vi "Reference Facade.vi"(0 "Data In":T4, 2 "Display State In":T2, 3 "Container State":T3) -> (6 "Data Out":T4, 7 "Display State Out":T2, 8 "Action":T1)   [LabVIEW 2016, in "VI Reference.xctl"]
uses:
  VI Reference.xctl
  Reference Data.ctl
  <vilib>/_xctls/Container State.ctl
  Reference State.ctl
  VI Reference Control/VI Reference Control.lvclass
  C:/Users/tblair/Documents/Git Projects/Drag and Drop VI Tool/Source/Reference Control/Reference Control.lvclass
  <vilib>/_xctls/Action.ctl
  <vilib>/Utility/miscctls.llb/LVRectTypeDef.ctl
  <vilib>/_xctls/XControlSupport.lvlib
  Reference Control/Reference Control.lvclass
panel:
  in  "Source Path":path
  out "Source Picture":picture
  # "1. Drop the controls that make up the appearance\nof the XControl here.\n\n2. Resize the window to fit the controls\n\n3. If the XControl is of fixed size,  make the \n window not resizable from VI Properties->Window Appearance.\n\n4. If you want the controls to automatically size when the XControl sizes, check  \"Scale all objects on front panel when window resizes\" in File->VI Properties->Window Size page.\n\n5. Show the block diagram and handle events for the controls on this panel."
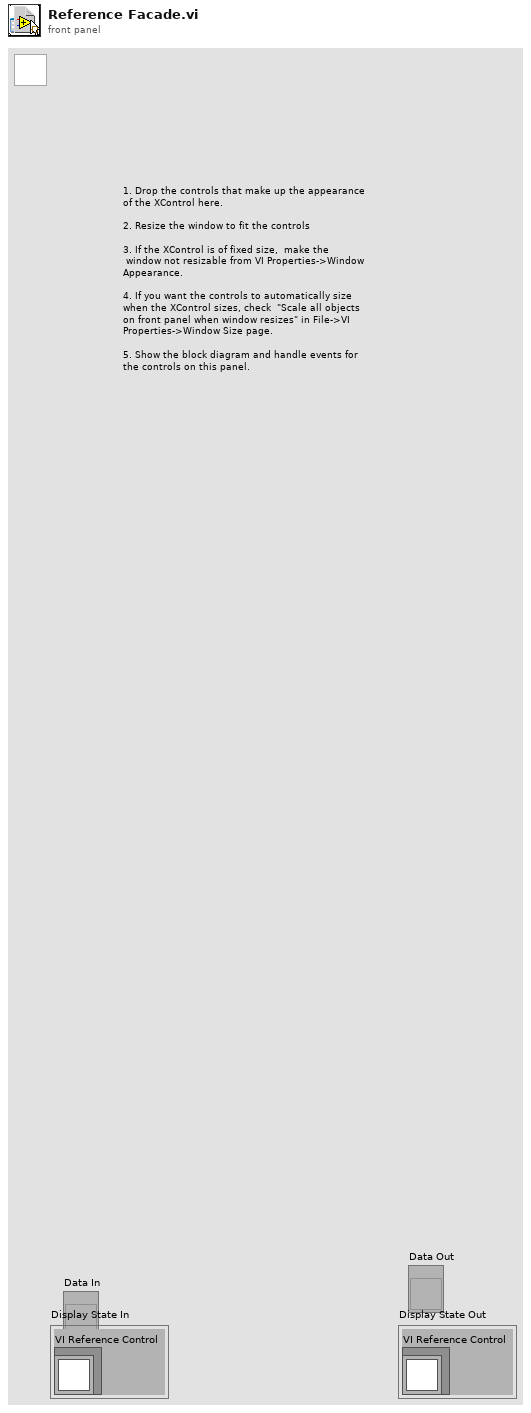
[diagram p1: front panel]
types:
  T1 = typedef "XControlSupport.lvlib/Action.ctl" = cluster{"Data Changed?":bool, "State Changed?":bool, "Action Name":string}
  T2 = typedef "VI Reference.xctl/Reference State.ctl" = cluster{"VI Reference Control":refnum<class "VI Reference Control.lvclass">}
  T3 = typedef "XControlSupport.lvlib/Container State.ctl" = cluster{"Indicator?":bool, "Run Mode?":bool, " Refnum":refnum<vi>}
  T4 = typedef "VI Reference.xctl/Reference Data.ctl" = refnum<vi>
  T5 = typedef "LVRectTypeDef.ctl" = cluster{"Left":i16, "Top":i16, "Right":i16, "Bottom":i16}
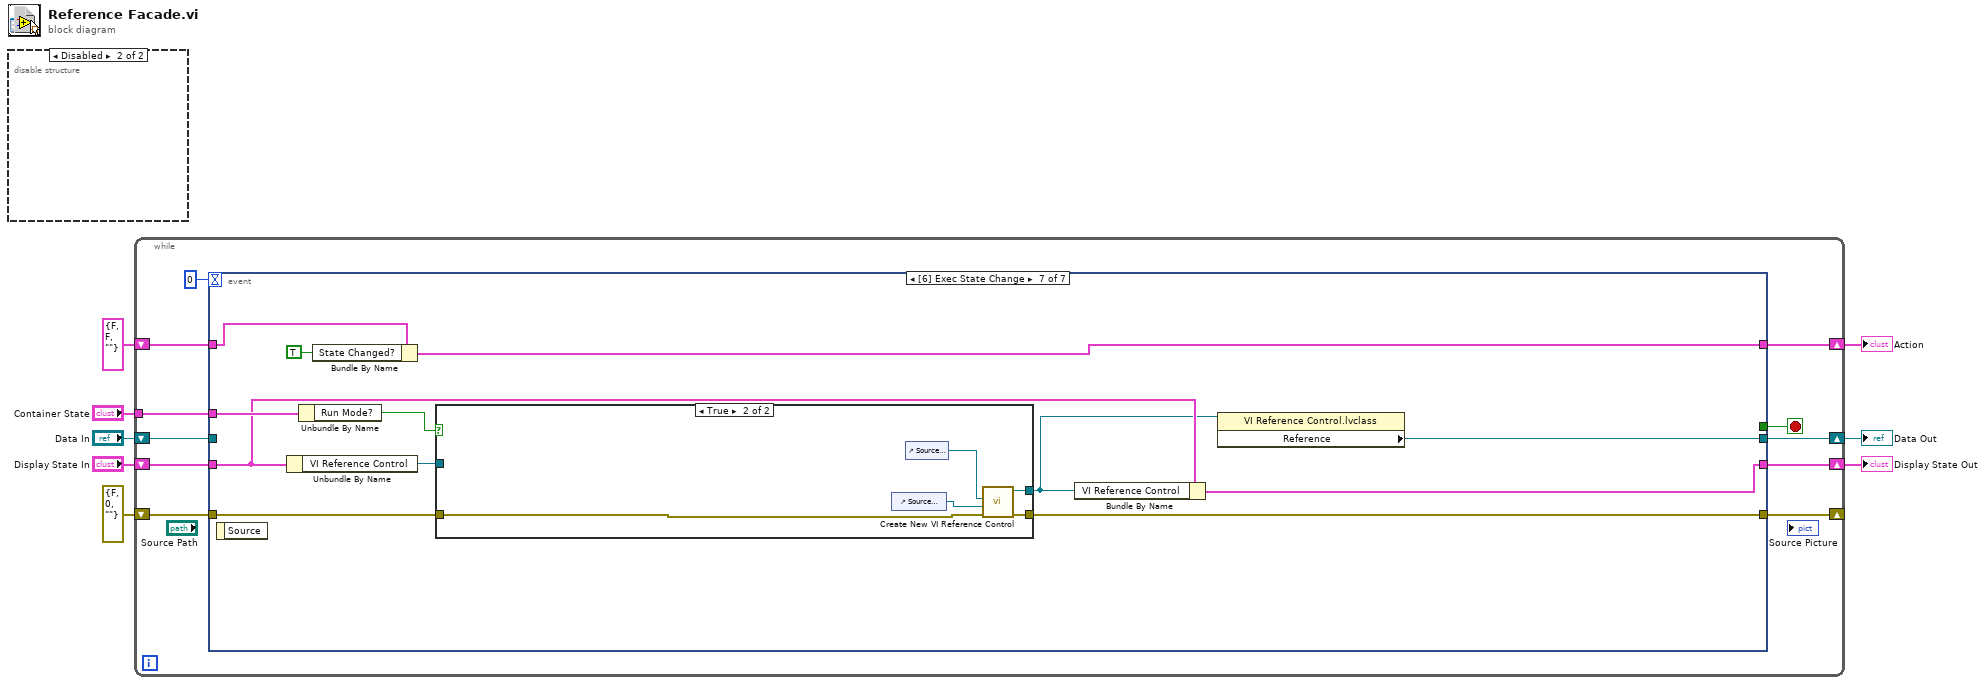
[diagram p0: block diagram]
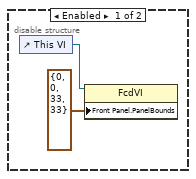
[diagram p2: hidden frame]
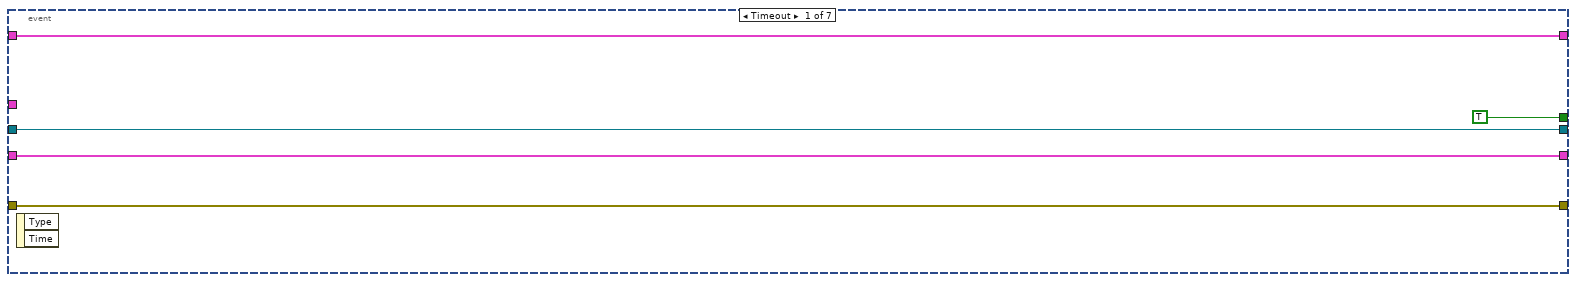
[diagram p3: hidden frame]
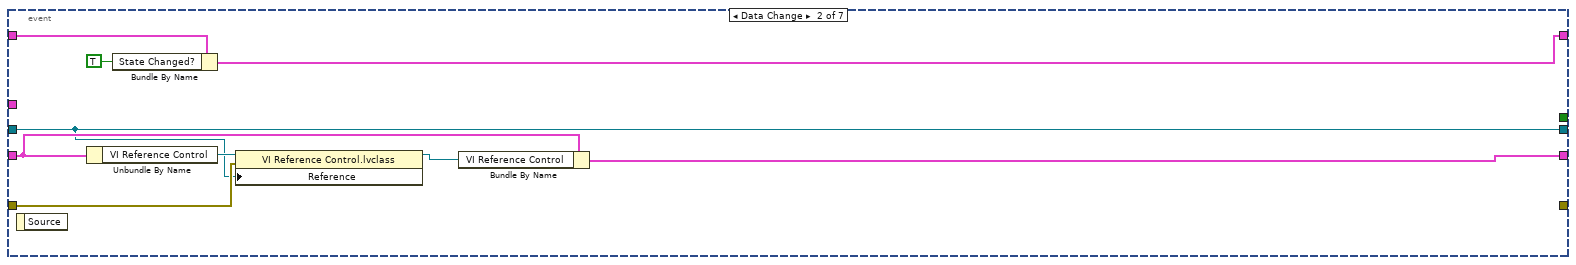
[diagram p4: hidden frame]
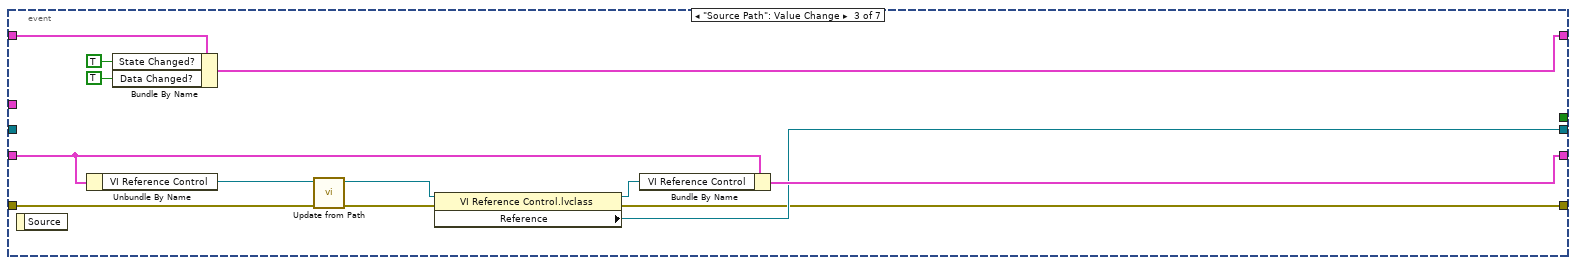
[diagram p5: hidden frame]
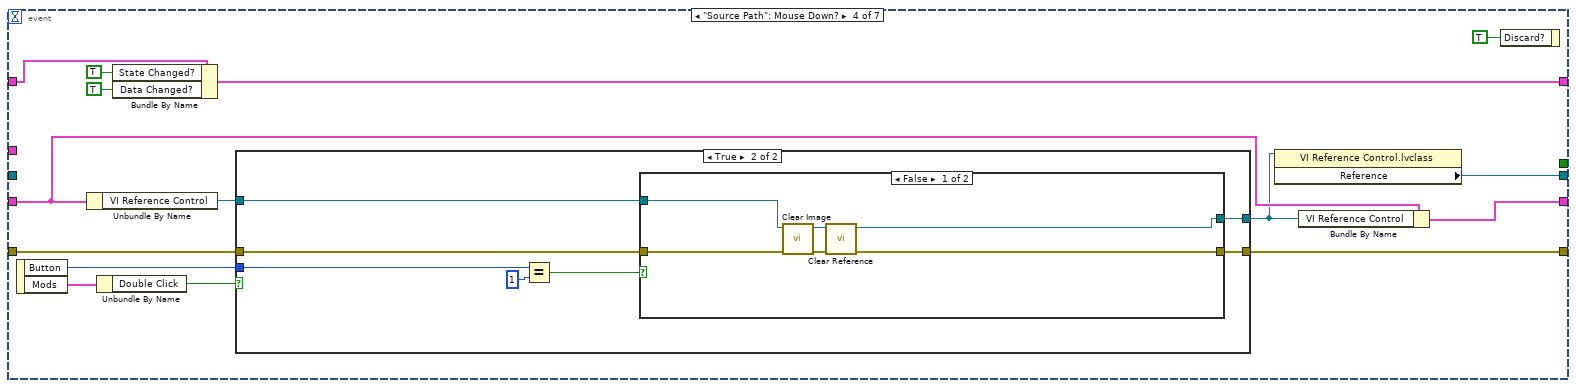
[diagram p6: hidden frame]
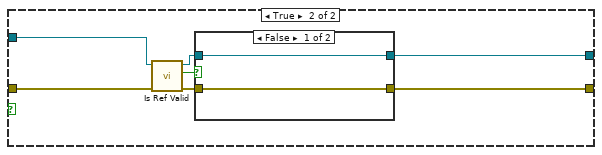
[diagram p8: hidden frame]
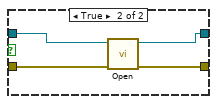
[diagram p9: hidden frame]
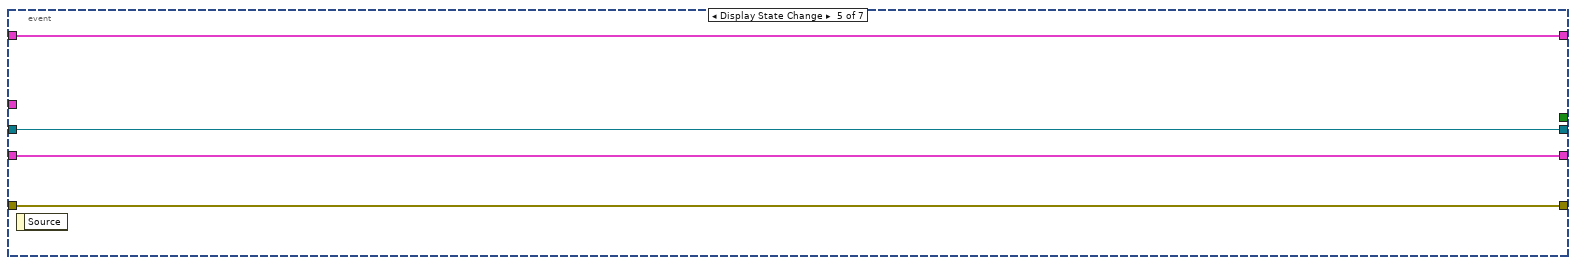
[diagram p10: hidden frame]
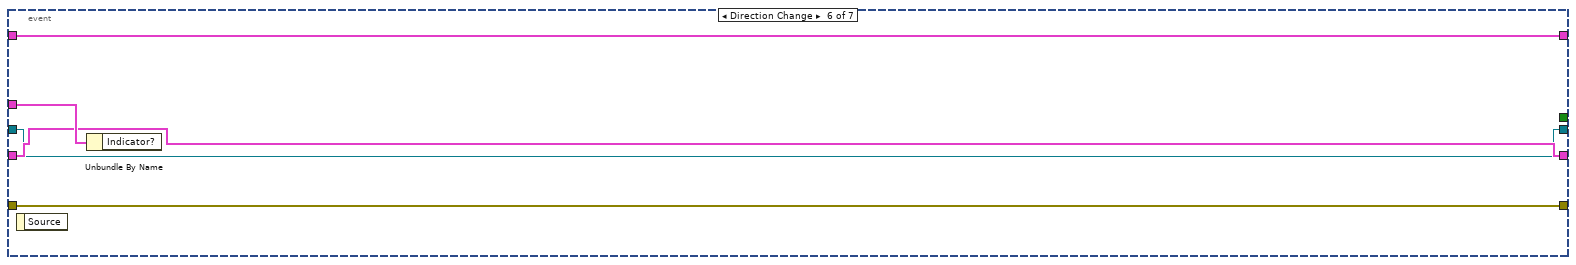
[diagram p11: hidden frame]
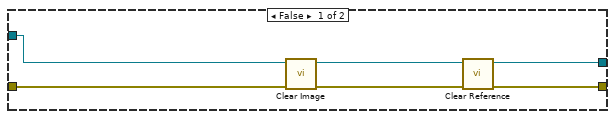
[diagram p12: hidden frame]
diagram:
  n1 = disable-structure shown="Disabled" {
    frame Enabled {
      n2 = control-ref of="This VI"() -> (w9:refnum<vi>)
      n3 = property class="FcdVI"(reference=w9, "Front Panel.PanelBounds"=T5 {"Left"=0, "Top"=0, "Right"=33, "Bottom"=33} ("Front Panel Window:Panel Bounds")) -> ()  [unwired: 1 in, 2 out]
    }
    frame Disabled {
    }
  }
  n4 = while {
    shift-right: [w20] -> w6
    shift-left: "Display State In" -> [w21]
    tunnel: "Container State" -> [w17]
    shift-right: [w15] -> w1
    shift-left: "Data In" -> [w16]
    shift-right: [w13] -> w4
    shift-left: T1 {"Data Changed?"=FALSE, "State Changed?"=FALSE, "Action Name"=""} ("Action") -> [w14]
    shift-right: [w12] -> _
    shift-left: errorcluster {"status"=FALSE, "code"=0, "source"=""} ("error out") -> [w11]
    stop <- w19 stop-if-true
    n5 = event shown="[6] Exec State Change" {
      selector: _ -> [_ _ _ _ _ _ _]
      dyn-events: _ -> [_ _ _ _ _ _ _]
      timeout: 0 -> [_ _ _ _ _ _ _]
      tunnel: w21 -> [w24 w34 w43 w56 w92 w99 w106]
      tunnel: [w24 w33 w42 w55 w92 w99 w101] -> w20
      tunnel: [TRUE _ _ _ _ _ _] -> w19
      tunnel: w17 -> [_ _ _ _ _ w100 w112]
      tunnel: w16 -> [w23 w31 _ _ w94 w98 _]
      tunnel: [w23 w31 w39 w51 w94 w98 w102] -> w15
      tunnel: [w25 w27 w46 w53 w93 w97 w107] -> w13
      tunnel: w14 -> [w25 w29 w47 w54 w93 w97 w108]
      tunnel: [w22 _ w36 w59 w95 w96 w109] -> w12
      tunnel: w11 -> [w22 w35 w48 w60 w95 w96 w110]
      event Timeout {
        n6 = event-data() -> ()  [unwired: 1 in, 2 out]
      }
      event Data Change {
        n7 = event-data() -> ()  [unwired: 1 in, 1 out]
        n8 = Unbundle By Name(w34) -> ("VI Reference Control"=w32:refnum<class "VI Reference Control.lvclass">)
        n9 = Bundle By Name(cluster=w29, "State Changed?"=TRUE) -> (w27:T1)
        n10 = property class="VI Reference Control.lvclass"(reference=w32, error in=w35, "Reference"=w31) -> (reference out=w30:refnum<class "VI Reference Control.lvclass">)  [unwired: 1 out]
        n11 = Bundle By Name(cluster=w34, "VI Reference Control"=w30) -> (w33:T2)
      }
      event "Source Path": Value Change {
        n12 = event-data() -> ()  [unwired: 1 in, 1 out]
        n13 = Unbundle By Name(w43) -> ("VI Reference Control"=w44:refnum<class "VI Reference Control.lvclass">)
        n14 = Bundle By Name(cluster=w47, "State Changed?"=TRUE ("Data Changed?"), "Data Changed?"=TRUE) -> (w46:T1)
        n15 = call "Update from Path.vi"("error in (no error)"=w48, "Reference Control in"=w44) -> ("error out"=w37:errorcluster, "Reference Control out"=w40:refnum<class "VI Reference Control.lvclass">)  [unwired: 8 in]
        n16 = property class="VI Reference Control.lvclass"(reference=w40, error in=w37) -> (reference out=w38:refnum<class "VI Reference Control.lvclass">, error out=w36:errorcluster, "Reference"=w39:refnum<vi>)
        n17 = Bundle By Name(cluster=w43, "VI Reference Control"=w38) -> (w42:T2)
      }
      event "Source Path": Mouse Down? {
        n18 = event-data() -> ("Button"=w61:u16, "Mods"=w62:cluster{"Double Click":bool, "Menu Key":bool})  [unwired: 1 in]
        n19 = Unbundle By Name(w56) -> ("VI Reference Control"=w57:refnum<class "VI Reference Control.lvclass">)
        n20 = Unbundle By Name(w62) -> ("Double Click"=w63:bool)
        n21 = Bundle By Name(cluster=w54, "State Changed?"=TRUE, "Data Changed?"=TRUE) -> (w53:T1)
        n22 = case shown="True" w63 {
          tunnel: w61 -> [_ w70]
          tunnel: w57 -> [w65 w69]
          tunnel: [w65 w68] -> w52
          tunnel: w60 -> [w64 w67]
          tunnel: [w64 w66] -> w59
          frame False {
          }
          frame True {
            n23 = Equal?(x=w70, y=u16 1) -> (x = y?=w71:bool)
            n24 = case shown="False" w71 {
              tunnel: w69 -> [w77 w84]
              tunnel: [w78 w85] -> w68
              tunnel: w67 -> [w75 w81]
              tunnel: [w73 w79] -> w66
              frame False {
                n25 = call "Clear Image.vi"("error in (no error)"=w75, "Reference Control in"=w77) -> ("error out"=w74:errorcluster, "Reference Control out"=w76:refnum<class "VI Reference Control.lvclass">)  [unwired: 8 in]
                n26 = call-dynamic "Clear Reference.vi"("error in (no error)"=w74, "VI Reference Control in"=w76) -> ("error out"=w73:errorcluster, "VI Reference Control out"=w78:refnum<class "VI Reference Control.lvclass">)  [unwired: 8 in]
              }
              frame True {
                n27 = call-dynamic "Is Ref Valid.vi"("error in (no error)"=w81, "VI Reference Control in"=w84) -> ("error out"=w80:errorcluster, "Refnum Valid?"=w83:bool, "VI Reference Control out"=w82:refnum<class "VI Reference Control.lvclass">)  [unwired: 7 in]
                n28 = case shown="False" w83 {
                  tunnel: w82 -> [w87 w91]
                  tunnel: [w87 w90] -> w85
                  tunnel: w80 -> [w86 w89]
                  tunnel: [w86 w88] -> w79
                  frame False {
                  }
                  frame True {
                    n29 = call-dynamic "Open.vi"("error in (no error)"=w89, "VI Reference Control in"=w91) -> ("error out"=w88:errorcluster, "VI Reference Control out"=w90:refnum<class "VI Reference Control.lvclass">)  [unwired: 8 in]
                  }
                }
              }
            }
          }
        }
        n30 = property class="VI Reference Control.lvclass"(reference=w52) -> ("Reference"=w51:refnum<vi>)  [unwired: 1 in, 2 out]
        n31 = Bundle By Name(cluster=w56, "VI Reference Control"=w52) -> (w55:T2)
        n32 = event-data("Discard?"=TRUE) -> ()  [unwired: 1 in, 1 out]
      }
      event Display State Change {
        n33 = event-data() -> ()  [unwired: 1 in, 1 out]
      }
      event Direction Change {
        n34 = event-data() -> ()  [unwired: 1 in, 1 out]
        n35 = Unbundle By Name(w100) -> ()  [unwired: 1 out]
      }
      event Exec State Change {
        n36 = event-data() -> ()  [unwired: 1 in, 1 out]
        n37 = Unbundle By Name(w106) -> ("VI Reference Control"=w105:refnum<class "VI Reference Control.lvclass">)
        n38 = Unbundle By Name(w112) -> ("Run Mode?"=w111:bool)
        n39 = Bundle By Name(cluster=w108, "State Changed?"=TRUE) -> (w107:T1)
        n40 = case shown="True" w111 {
          tunnel: w105 -> [w116 _]
          tunnel: [w118 w121] -> w103
          tunnel: w110 -> [w114 w120]
          tunnel: [w117 w119] -> w109
          frame False {
            n41 = call "Clear Image.vi"("error in (no error)"=w114, "Reference Control in"=w116) -> ("error out"=w113:errorcluster, "Reference Control out"=w115:refnum<class "VI Reference Control.lvclass">)  [unwired: 8 in]
            n42 = call-dynamic "Clear Reference.vi"("error in (no error)"=w113, "VI Reference Control in"=w115) -> ("error out"=w117:errorcluster, "VI Reference Control out"=w118:refnum<class "VI Reference Control.lvclass">)  [unwired: 8 in]
          }
          frame True {
            n43 = control-ref of="Source Picture"() -> (w122:refnum<vi>)
            n44 = control-ref of="Source Path"() -> (w123:refnum<vi>)
            n45 = call "Create New VI Reference Control.vi"("error in (no error)"=w120, "Picture Control Ref"=w122, "Path Control Ref"=w123) -> ("error out"=w119:errorcluster, "VI Reference Control out"=w121:refnum<class "VI Reference Control.lvclass">)  [unwired: 7 in]
          }
        }
        n46 = Bundle By Name(cluster=w106, "VI Reference Control"=w103) -> (w101:T2)
        n47 = property class="VI Reference Control.lvclass"(reference=w103) -> ("Reference"=w102:refnum<vi>)  [unwired: 1 in, 2 out]
      }
    }
  }
  "Display State Out" <- w6
  "Data Out" <- w1
  "Action" <- w4
